vi "Refresh Panels.vi"(11 "Entity Editor in":refnum<class "Entity Editor.lvclass">) -> (3 "Entity Editor out":refnum<class "Entity Editor.lvclass">)   [LabVIEW 2020, in "Conditum-Tools.lvlib" / "Entity Editor.lvclass"]
uses:
  Entity Editor.lvclass
  Entity Editor.lvclass/Entity Editor.ctl
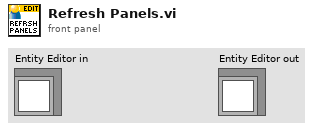
[diagram p1: front panel]
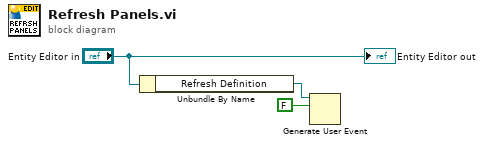
[diagram p0: block diagram]
diagram:
  n1 = Unbundle By Name("Entity Editor in") -> ("Refresh Definition"=w2:refnum<user-event>)
  n2 = Generate User Event(user event=w2, event data cluster=FALSE ("event data")) -> ()  [unwired: 2 in, 2 out]
  "Entity Editor out" <- "Entity Editor in"
